vi "First Ex.vi"() -> ()   [LabVIEW 2016]
panel:
  in  "stop":bool
  out "Boolean 3":bool
  out "Boolean 2":bool
  in  "Boolean":bool
  out "Meter":dbl(knob) scale=0.0..10.0
  out "Numeric 2":dbl
  in  "Numeric":dbl
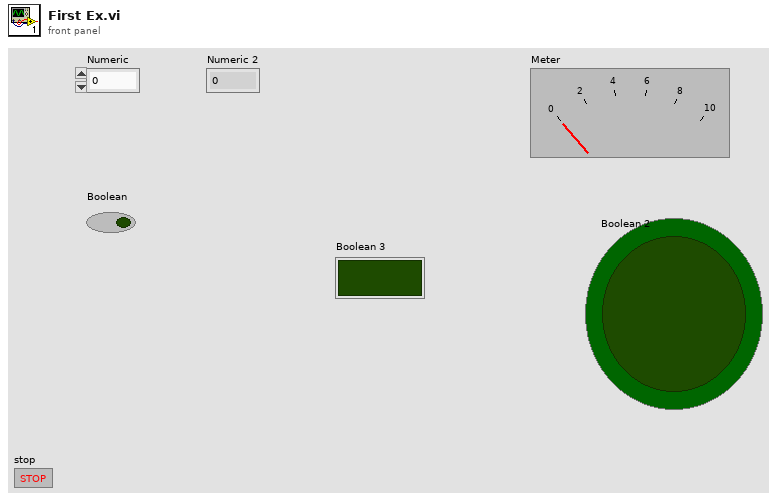
[diagram p1: front panel]
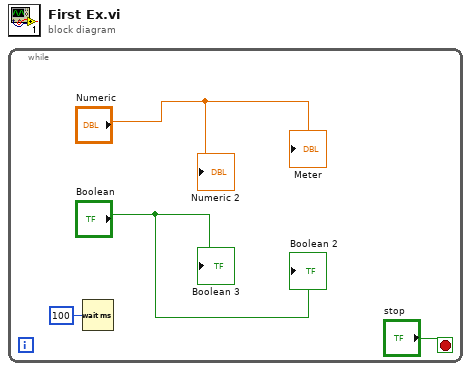
[diagram p0: block diagram]
diagram:
  n1 = while {
    stop <- "stop" stop-if-true
    n2 = Wait (ms)(milliseconds to wait=u32 100) -> ()  [unwired: 1 out]
    "Numeric 2" <- "Numeric"
    "Meter" <- "Numeric"
    "Boolean 2" <- "Boolean"
    "Boolean 3" <- "Boolean"
  }
